vi "Get cif_manager_PluginInfoResponse.vi"(8 "error in (no error)":errorcluster, 11 "gRPCid":T1) -> (0 "error out":errorcluster, 2 "package_templatemessage":T2, 3 "gRPCid out":T1)   [LabVIEW 2021, in "CIF_PluginLoader_server.lvlib"]
uses:
  CIF_PluginLoader_server.lvlib
  cif_manager_PluginInfoResponse.ctl
  cif_manager_PluginInfo.ctl
  cif_common_ShortVersion.ctl
  cif_plugincore_StatusData.ctl
  cif_plugincore_StatusData_PluginState.ctl
  cif_plugincore_TimingStatistics.ctl
  cif_common_TimingStats.ctl
  cif_plugincore_FifoStatistics.ctl
  cif_plugincore_Error.ctl
  cif_plugincore_MonitorDoubles.ctl
  cif_plugincore_MonitorU64.ctl
  cif_plugincore_MonitorI64.ctl
  cif_common_Status.ctl
  <vilib>/gRPC/LabVIEW gRPC Library/Shared/grpcId.ctl
  cif_manager_PluginInfoResponse_Flat.ctl
  cif_manager_PluginInfo_Flat.ctl
  cif_common_ShortVersion_Flat.ctl
  cif_plugincore_StatusData_Flat.ctl
  cif_plugincore_TimingStatistics_Flat.ctl
  cif_common_TimingStats_Flat.ctl
  cif_plugincore_FifoStatistics_Flat.ctl
  cif_plugincore_Error_Flat.ctl
  cif_plugincore_MonitorDoubles_Flat.ctl
  cif_plugincore_MonitorU64_Flat.ctl
  cif_plugincore_MonitorI64_Flat.ctl
  cif_common_Status_Flat.ctl
  2ed25e12-861d-4677-8ead-ace2906b2041.vi
  <vilib>/gRPC/LabVIEW gRPC Library/Shared/TranslateGrpcError.vi
  FlatToRichcif_manager_PluginInfo.vi
  FlatToRichcif_common_Status.vi
  FlatToRichcif_common_ShortVersion.vi
  FlatToRichcif_plugincore_StatusData.vi
  FlatToRichcif_plugincore_TimingStatistics.vi
  FlatToRichcif_plugincore_FifoStatistics.vi
  FlatToRichcif_plugincore_Error.vi
  FlatToRichcif_plugincore_MonitorDoubles.vi
  FlatToRichcif_plugincore_MonitorU64.vi
  FlatToRichcif_plugincore_MonitorI64.vi
  FlatToRichcif_common_TimingStats.vi
  <vilib>/gRPC/LabVIEW gRPC Library/Server API/Server/Get Server DLL Path.vi
  <vilib>/Utility/error.llb/Error Cluster From Error Code.vi
  <vilib>/gRPC/LabVIEW gRPC Library/grpc-lvsupport-release.lvlib
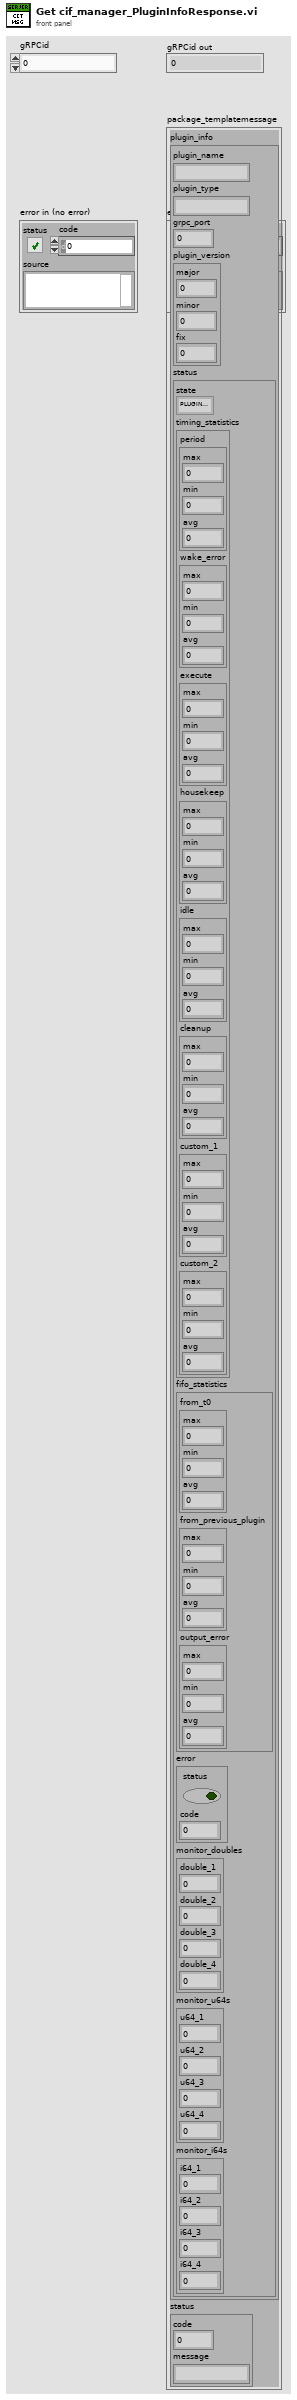
[diagram p1: front panel]
types:
  T1 = typedef "grpc-lvsupport-release.lvlib/grpcId.ctl" = u64
  T2 = typedef "CIF_PluginLoader_server.lvlib/cif_manager_PluginInfoResponse.ctl" = cluster{"plugin_info":T3, "status":T14}
  T3 = typedef "CIF_PluginLoader_server.lvlib/cif_manager_PluginInfo.ctl" = cluster{"plugin_name":string, "plugin_type":string, "grpc_port":i32, "plugin_version":T4, "status":T5}
  T4 = typedef "CIF_PluginLoader_server.lvlib/cif_common_ShortVersion.ctl" = cluster{"major":u32, "minor":u32, "fix":u32}
  T5 = typedef "CIF_PluginLoader_server.lvlib/cif_plugincore_StatusData.ctl" = cluster{"state":T6, "timing_statistics":T7, "fifo_statistics":T9, "error":T10, "monitor_doubles":T11, "monitor_u64s":T12, "monitor_i64s":T13}
  T6 = typedef "CIF_PluginLoader_server.lvlib/cif_plugincore_StatusData_PluginState.ctl" = enum32{"PLUGINSTATE_UNKNOWN", "PLUGINSTATE_CREATING", "PLUGINSTATE_LISTENING", "PLUGINSTATE_RUNNING", "PLUGINSTATE_CLEANINGUP", "PLUGINSTATE_DESTROYING"}
  T7 = typedef "CIF_PluginLoader_server.lvlib/cif_plugincore_TimingStatistics.ctl" = cluster{"period":T8, "wake_error":T8, "execute":T8, "housekeep":T8, "idle":T8, "cleanup":T8, "custom_1":T8, "custom_2":T8}
  T8 = typedef "CIF_PluginLoader_server.lvlib/cif_common_TimingStats.ctl" = cluster{"max":i64, "min":i64, "avg":dbl}
  T9 = typedef "CIF_PluginLoader_server.lvlib/cif_plugincore_FifoStatistics.ctl" = cluster{"from_t0":T8, "from_previous_plugin":T8, "output_error":T8}
  T10 = typedef "CIF_PluginLoader_server.lvlib/cif_plugincore_Error.ctl" = cluster{"status":bool, "code":i32}
  T11 = typedef "CIF_PluginLoader_server.lvlib/cif_plugincore_MonitorDoubles.ctl" = cluster{"double_1":dbl, "double_2":dbl, "double_3":dbl, "double_4":dbl}
  T12 = typedef "CIF_PluginLoader_server.lvlib/cif_plugincore_MonitorU64.ctl" = cluster{"u64_1":u64, "u64_2":u64, "u64_3":u64, "u64_4":u64}
  T13 = typedef "CIF_PluginLoader_server.lvlib/cif_plugincore_MonitorI64.ctl" = cluster{"i64_1":i64, "i64_2":i64, "i64_3":i64, "i64_4":i64}
  T14 = typedef "CIF_PluginLoader_server.lvlib/cif_common_Status.ctl" = cluster{"code":i32, "message":string}
  T15 = typedef "CIF_PluginLoader_server.lvlib/cif_manager_PluginInfoResponse_Flat.ctl" = cluster{"plugin_info":T16, "status":T26}
  T16 = typedef "CIF_PluginLoader_server.lvlib/cif_manager_PluginInfo_Flat.ctl" = cluster{"plugin_name":string, "plugin_type":string, "grpc_port":i32, "plugin_version":T17, "status":T18}
  T17 = typedef "CIF_PluginLoader_server.lvlib/cif_common_ShortVersion_Flat.ctl" = cluster{"major":u32, "minor":u32, "fix":u32}
  T18 = typedef "CIF_PluginLoader_server.lvlib/cif_plugincore_StatusData_Flat.ctl" = cluster{"state":T6, "timing_statistics":T19, "fifo_statistics":T21, "error":T22, "monitor_doubles":T23, "monitor_u64s":T24, "monitor_i64s":T25}
  T19 = typedef "CIF_PluginLoader_server.lvlib/cif_plugincore_TimingStatistics_Flat.ctl" = cluster{"period":T20, "wake_error":T20, "execute":T20, "housekeep":T20, "idle":T20, "cleanup":T20, "custom_1":T20, "custom_2":T20}
  T20 = typedef "CIF_PluginLoader_server.lvlib/cif_common_TimingStats_Flat.ctl" = cluster{"max":i64, "min":i64, "avg":dbl}
  T21 = typedef "CIF_PluginLoader_server.lvlib/cif_plugincore_FifoStatistics_Flat.ctl" = cluster{"from_t0":T20, "from_previous_plugin":T20, "output_error":T20}
  T22 = typedef "CIF_PluginLoader_server.lvlib/cif_plugincore_Error_Flat.ctl" = cluster{"status":bool, "code":i32}
  T23 = typedef "CIF_PluginLoader_server.lvlib/cif_plugincore_MonitorDoubles_Flat.ctl" = cluster{"double_1":dbl, "double_2":dbl, "double_3":dbl, "double_4":dbl}
  T24 = typedef "CIF_PluginLoader_server.lvlib/cif_plugincore_MonitorU64_Flat.ctl" = cluster{"u64_1":u64, "u64_2":u64, "u64_3":u64, "u64_4":u64}
  T25 = typedef "CIF_PluginLoader_server.lvlib/cif_plugincore_MonitorI64_Flat.ctl" = cluster{"i64_1":i64, "i64_2":i64, "i64_3":i64, "i64_4":i64}
  T26 = typedef "CIF_PluginLoader_server.lvlib/cif_common_Status_Flat.ctl" = cluster{"code":i32, "message":string}
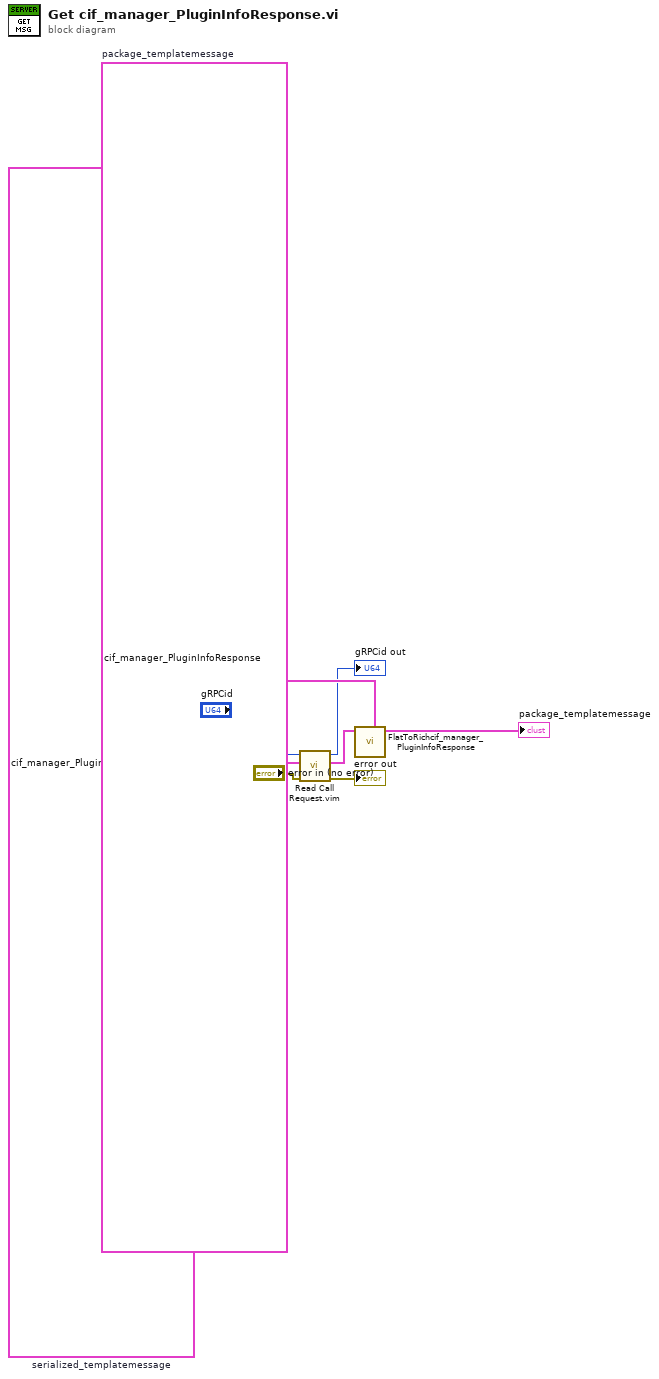
[diagram p0: block diagram]
diagram:
  w6 = T15 {"plugin_info"={"plugin_name"="", "plugin_type"="", "grpc_port"=0, "plugin_version"={"major"=0, "minor"=0, "fix"=0}, "status"={"state"=enum."PLUGINSTATE_UNKNOWN", "timing_statistics"={"period"={"max"=0, "min"=0, "avg"=0.0}, "wake_error"={"max"=0, "min"=0, "avg"=0.0}, "execute"={"max"=0, "min"=0, "avg"=0.0}, "housekeep"={"max"=0, "min"=0, "avg"=0.0}, "idle"={"max"=0, "min"=0, "avg"=0.0}, "cleanup"={"max"=0, "min"=0, "avg"=0.0}, "custom_1"={"max"=0, "min"=0, "avg"=0.0}, "custom_2"={"max"=0, "min"=0, "avg"=0.0}}, "fifo_statistics"={"from_t0"={"max"=0, "min"=0, "avg"=0.0}, "from_previous_plugin"={"max"=0, "min"=0, "avg"=0.0}, "output_error"={"max"=0, "min"=0, "avg"=0.0}}, "error"={"status"=FALSE, "code"=0}, "monitor_doubles"={"double_1"=0.0, "double_2"=0.0, "double_3"=0.0, "double_4"=0.0}, "monitor_u64s"={"u64_1"=0, "u64_2"=0, "u64_3"=0, "u64_4"=0}, "monitor_i64s"={"i64_1"=0, "i64_2"=0, "i64_3"=0, "i64_4"=0}}}, "status"={"code"=0, "message"=""}}  # serialized_templatemessage
  w5 = T2 {"plugin_info"={"plugin_name"="", "plugin_type"="", "grpc_port"=0, "plugin_version"={"major"=0, "minor"=0, "fix"=0}, "status"={"state"=enum."PLUGINSTATE_UNKNOWN", "timing_statistics"={"period"={"max"=0, "min"=0, "avg"=0.0}, "wake_error"={"max"=0, "min"=0, "avg"=0.0}, "execute"={"max"=0, "min"=0, "avg"=0.0}, "housekeep"={"max"=0, "min"=0, "avg"=0.0}, "idle"={"max"=0, "min"=0, "avg"=0.0}, "cleanup"={"max"=0, "min"=0, "avg"=0.0}, "custom_1"={"max"=0, "min"=0, "avg"=0.0}, "custom_2"={"max"=0, "min"=0, "avg"=0.0}}, "fifo_statistics"={"from_t0"={"max"=0, "min"=0, "avg"=0.0}, "from_previous_plugin"={"max"=0, "min"=0, "avg"=0.0}, "output_error"={"max"=0, "min"=0, "avg"=0.0}}, "error"={"status"=FALSE, "code"=0}, "monitor_doubles"={"double_1"=0.0, "double_2"=0.0, "double_3"=0.0, "double_4"=0.0}, "monitor_u64s"={"u64_1"=0, "u64_2"=0, "u64_3"=0, "u64_4"=0}, "monitor_i64s"={"i64_1"=0, "i64_2"=0, "i64_3"=0, "i64_4"=0}}}, "status"={"code"=0, "message"=""}}  # package_templatemessage
  n1 = call "Read Call Request.vim"("error in"="error in (no error)", "Request Type"=w6, "gRPCid in"="gRPCid") -> ("error out"=→"error out":errorcluster, "Request Data"=w4:T15, "gRPCid out"=→"gRPCid out":T1)  [unwired: 6 in]
  n2 = call "FlatToRichcif_manager_PluginInfoResponse.vi"("OutputClusterType"=w5, "InputCluster"=w4) -> ("OutputCluster"=→"package_templatemessage":T2)  [unwired: 9 in]
